vi "Load one U16 Image with metadata from Tiff Stack file.vi"(7 "path to TIFF file":path=path "/HD1/Users/herbertlooser/Desktop/LadungssprŸher.tif", 8 "error in":errorcluster, 10 "Index of image\n to read":i32, 11 "U16 Image":T1) -> (0 "error out":errorcluster, 3 "U16 Image dup":T1)   [LabVIEW 2013, in "Tiff reader.lvlib"]
doc: "This .vi is taken from an online tiff reader. It is able to read 32-bit floating point .tiff images."
uses:
  Tiff reader.lvlib
  <vilib>/vision/Image Controls.llb/IMAQ Image.ctl
panel:
  out "Custom Data":string[](array[string])
  out "Keys":string[](array[string])
  out "U16":u16[][](array[numeric])
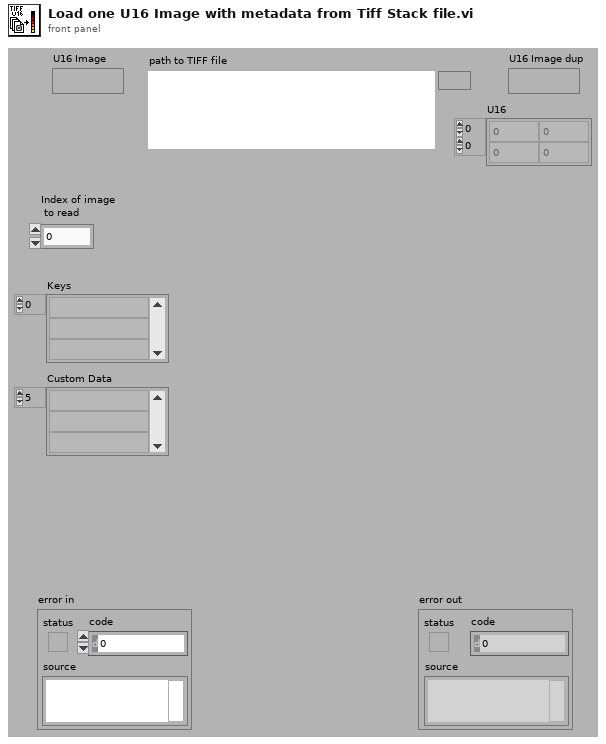
[diagram p1: front panel]
types:
  T1 = typedef "IMAQ Image.ctl" = refnum<image>
  T2 = enum16{"open", "replace", "create", "open or create", "replace or create", "replace or create with confirmation"}
  T3 = typedef "Tiff reader.lvlib/IFD Entry.ctl" = cluster{"Tag":u16, "Type":T4, "Count":u32, "Val/Offs":u32, "Is Pointer?":bool, "Byte stream index":i32}
  T4 = typedef "Tiff reader.lvlib/FieldTypes.ctl" = enum16{"NULL", "U8", "ASCII7", "U16", "U32", "RATIONAL", "SByte(I8)", "Undef(8Bit)", "I16", "I32", "SRat(4B:4B)", "SGL(4Byte)", "DBL(8Byte)"}
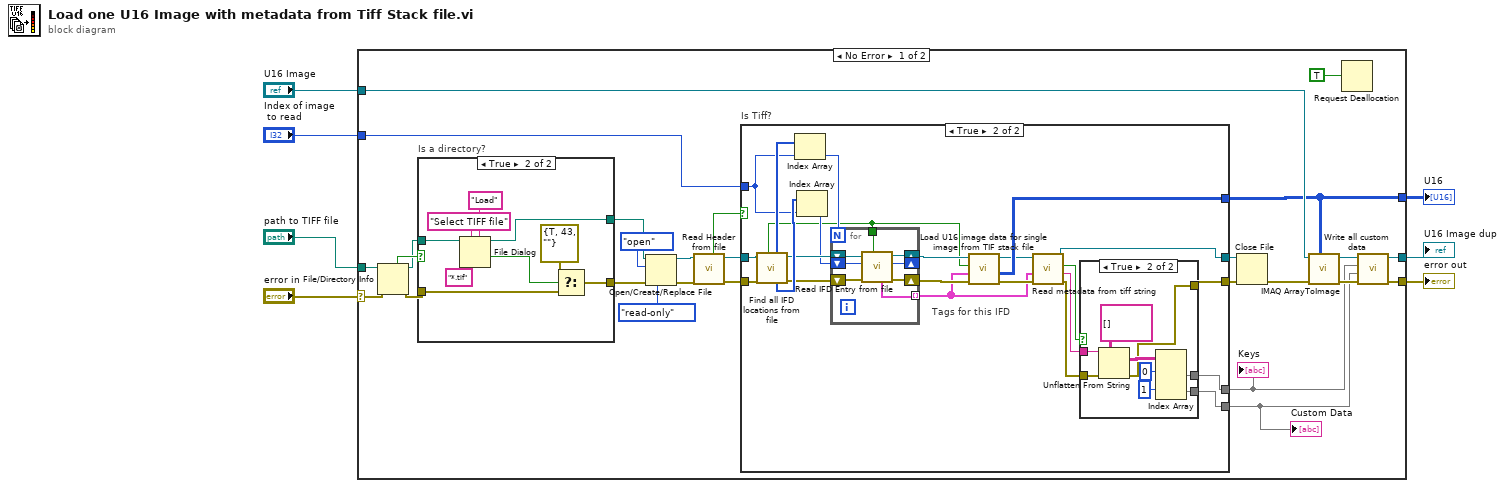
[diagram p0: block diagram]
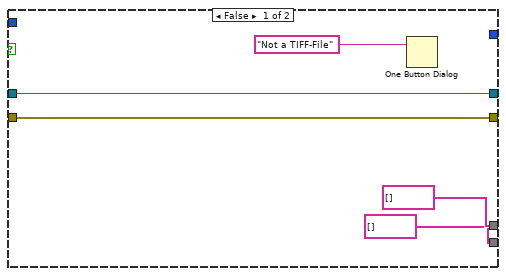
[diagram p2: hidden frame]
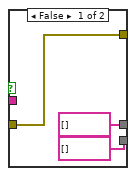
[diagram p3: hidden frame]
diagram:
  n1 = case shown="No Error" "error in" {
    selector: "error in" -> [w12 w95]
    tunnel: "path to TIFF file" -> [w33 _]
    tunnel: "Index of image\n to read" -> [w21 _]
    tunnel: [w8 _] -> w5
    tunnel: [w16 w94] -> w4
    tunnel: [w15 w95] -> w3
    tunnel: "U16 Image" -> [w11 w94]
    frame No Error {
      n2 = File/Directory Info(path=w33, error in=w12) -> (path out=w9:path, directory=w34:bool, error out=w32:errorcluster)  [unwired: 4 out]
      n3 = case "Is a directory?" shown="True" w34 {
        tunnel: w32 -> [w84 w90]
        tunnel: w9 -> [w83 w89]
        tunnel: [w84 w85] -> w24
        tunnel: [w83 w86] -> w23
        frame False {
        }
        frame True {
          n4 = File Dialog(5:"Load" ("button label"), 6:"*.tif" ("pattern"), 7:"Select TIFF file" ("prompt"), 11:w89) -> (1:w91:bool, 3:w86:path)  [unwired: 1 in, 4 out]
          n5 = Select(t=errorcluster {"status"=TRUE, "code"=43, "source"=""} ("error in (no error)"), s=w91, f=w90) -> (s? t:f=w85:errorcluster)
        }
      }
      n6 = Open/Create/Replace File(file path (use dialog)=w23, error in=w24, operation (0:open)=T2."open", access (0:read/write)=enum16{"read/write", "read-only", "write-only"}."read-only") -> (refnum out=w22:refnum<file>, error out=w25:errorcluster)  [unwired: 3 out]
      n7 = call "Read Header from file.vi"("error in"=w25, "File"=w22) -> ("error out"=w29:errorcluster, "File"=w28:refnum<file>, "isTIFF"=w30:bool)  [unwired: 5 out]
      n8 = case "Is Tiff?" shown="True" w30 {
        tunnel: w29 -> [w37 w54]
        tunnel: w28 -> [w38 w55]
        tunnel: [_ w45] -> w8
        tunnel: [w37 w56] -> w19
        tunnel: [w38 w62] -> w18
        tunnel: w21 -> [_ w40]
        tunnel: [string[] [] w59] -> w13
        tunnel: [string[] [] w58] -> w10
        frame False {
          n9 = One Button Dialog(message="Not a TIFF-File") -> ()  [unwired: 2 out]
        }
        frame True {
          # "Tags for this IFD"
          n10 = call "Find all IFD locations from file.vi"("error in"=w54, "File"=w55) -> ("error out"=w50:errorcluster, "File"=w52:refnum<file>, "1st tag locations"=w53:u32[], "# of tags in each IFD"=w49:u16[], "Litt/BigEnd"=w42:bool)  [unwired: 5 out]
          n11 = Index Array(array=w49, index=w40) -> (element=w48:u16)
          n12 = Index Array(array=w53, index=w40) -> (element=w51:u32)
          n13 = for {
            N: w48 -> [_]
            shift-right: [w65] -> w43
            shift-left: w52 -> [w70]
            shift-right: [w66] -> _
            shift-left: w51 -> [w67]
            tunnel: [w63] -> w41 mode=indexing
            tunnel: w42 -> [w64]
            shift-right: [w68] -> w47
            shift-left: w50 -> [w69]
            n14 = call "Read IFD Entry from file.vi"("Litt/BigEnd"=w64, "error in"=w69, "Tag location in"=w67, "File"=w70) -> ("error out"=w68:errorcluster, "Next Tag location Out\n(IN + 12)"=w66:i64, "File"=w65:refnum<file>, "Tag"=w63:T3)  [unwired: 1 in, 3 out]
          }
          n15 = call "Load U16 image data for single image from TIF stack file.vi"("error in"=w47, "DirEntries"=w41, "Litt/BigEnd"=w42, "File"=w43) -> ("error out"=w46:errorcluster, "U16"=w45:u16[][], "File"=w44:refnum<file>)  [unwired: 5 in]
          n16 = call "Read metadata from tiff string.vi"("error in"=w46, "DirEntries"=w41, "Tiff image stack"=w44) -> ("error out"=w60:errorcluster, "Metadata string"=w61:string, "Tag exists?"=w57:bool, "Tiff image stack dup"=w62:refnum<file>)  [unwired: 1 in, 4 out]
          n17 = case shown="True" w57 {
            tunnel: w61 -> [_ w82]
            tunnel: w60 -> [w73 w80]
            tunnel: [string[] [] w78] -> w59
            tunnel: [string[] [] w77] -> w58
            tunnel: [w73 w74] -> w56
            frame False {
            }
            frame True {
              n18 = Unflatten From String(type=string[][] [], binary string=w82, error in (no error)=w80) -> (value=w79:string[][], error out=w74:errorcluster)  [unwired: 3 out]
              n19 = Index Array(array=w79, index (row) #1=0 ("index (row)"), index (row) #2=1 ("index (row)")) -> (element #1=w78:string[], element #2=w77:string[])  [unwired: 2 in]
            }
          }
        }
      }
      "Keys" <- w13
      "Custom Data" <- w10
      n20 = Close File(refnum=w18, error in=w19) -> (error out=w20:errorcluster)  [unwired: 1 out]
      n21 = call "IMAQ ArrayToImage"("Image Pixels (U16)"=w8, "error in (no error)"=w20, "Image"=w11) -> ("error out"=w14:errorcluster, "Image Out"=w17:T1)  [unwired: 3 in, 4 out]
      n22 = Request Deallocation(TRUE ("flag")) -> ()
      n23 = call "Write all custom data.vi"("error in (no error)"=w14, "Custom Data"=w10, "Keys"=w13, "img"=w17) -> ("error out"=w15:errorcluster, "Image (duplicate)"=w16:T1)  [unwired: 6 out]
    }
    frame Error {
    }
  }
  "error out" <- w3
  "U16" <- w5
  "U16 Image dup" <- w4
